vi "arduino Motor Control Driver Read Position.vi"(8 "error in (no error)":errorcluster, 10 "Motor ID":u16 max=3 step=1, 11 "Port In":refnum<visa-resource-name>) -> (0 "error out":errorcluster, 1 "Position":i32, 2 "Motor ID dup":u16 max=3 step=1, 3 "Port Out":refnum<visa-resource-name>)   [LabVIEW 2019]
panel:
  out "Raw Response":string
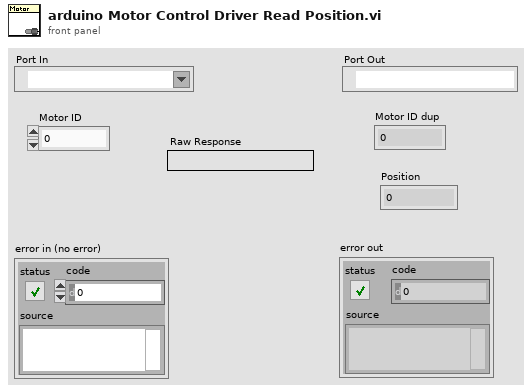
[diagram p1: front panel]
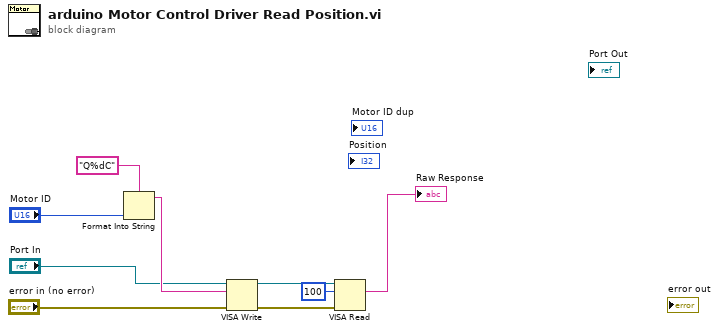
[diagram p0: block diagram]
diagram:
  n1 = Format Into String(format string="Q%dC", "Motor ID") -> (resulting string=w7:string)  [unwired: 2 in, 1 out]
  n2 = VISA Write(VISA resource name="Port In", write buffer=w7, error in (no error)="error in (no error)") -> (VISA resource name out=w3:refnum<visa-resource-name>, error out=w4:errorcluster)  [unwired: 1 out]
  n3 = VISA Read(VISA resource name=w3, byte count=u32 100, error in (no error)=w4) -> (read buffer=→"Raw Response":string)  [unwired: 3 out]
